vi "Convert to RelativePath.vi"(8 "error in (no error)":errorcluster caption="错误输入（无错误）", 11 "VI Path":path) -> (0 "error out":errorcluster caption="错误输出", 3 "RelativePath":string)   [LabVIEW 2013, in "PanelRootNode.lvclass"]
uses:
  PanelRootNode.lvclass
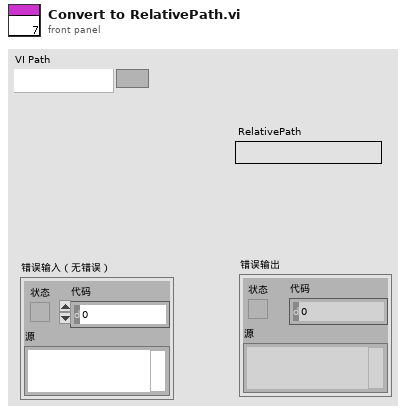
[diagram p1: front panel]
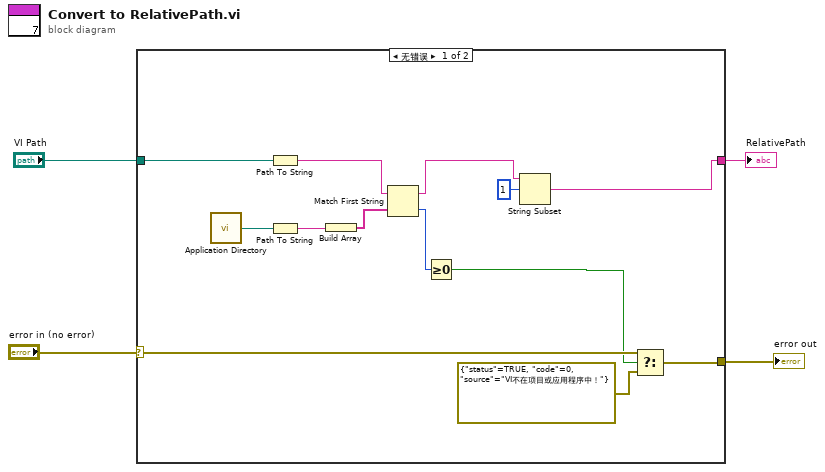
[diagram p0: block diagram]
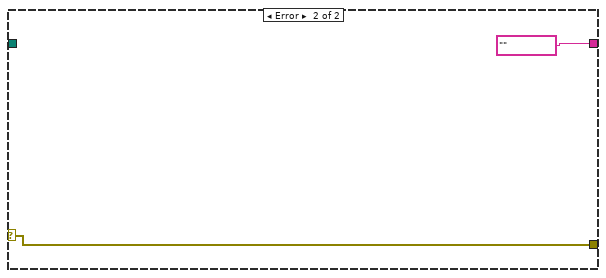
[diagram p2: hidden frame]
diagram:
  n1 = case shown="无错误" "error in (no error)" {
    selector: "error in (no error)" -> [w15 w19]
    tunnel: [w16 w19] -> w4
    tunnel: "VI Path" -> [w14 _]
    tunnel: [w6 ""] -> w1
    frame No Error {
      n2 = call <vilib>:"Application Directory.vi"() -> ("Application Directory"=w13:path)
      n3 = Path To String(path=w14) -> (string=w11:string)
      n4 = Path To String(path=w13) -> (string=w10:string)
      n5 = Build Array(w10) -> (w9:string[])
      n6 = Match First String(2:w9, 3:w11) -> (0:w8:i32, 1:w7:string)
      n7 = Greater Or Equal To 0?(x=w8) -> (x >= 0?=w12:bool)
      n8 = String Subset(string=w7, offset (0)=1 ("偏移量(0)")) -> (substring=w6:string)  [unwired: 1 in]
      n9 = Select(t=w15, s=w12, f=errorcluster {"status"=TRUE, "code"=0, "source"="VI不在项目或应用程序中！"}) -> (s? t:f=w16:errorcluster)
    }
    frame Error {
    }
  }
  "error out" <- w4
  "RelativePath" <- w1
